vi "ex10.vi"() -> ()   [LabVIEW 2025]
panel:
  out "impairs":i32[](array[numeric])
  out "pair":i32[](array[numeric])
  in  "input":i32[][](array[numeric])
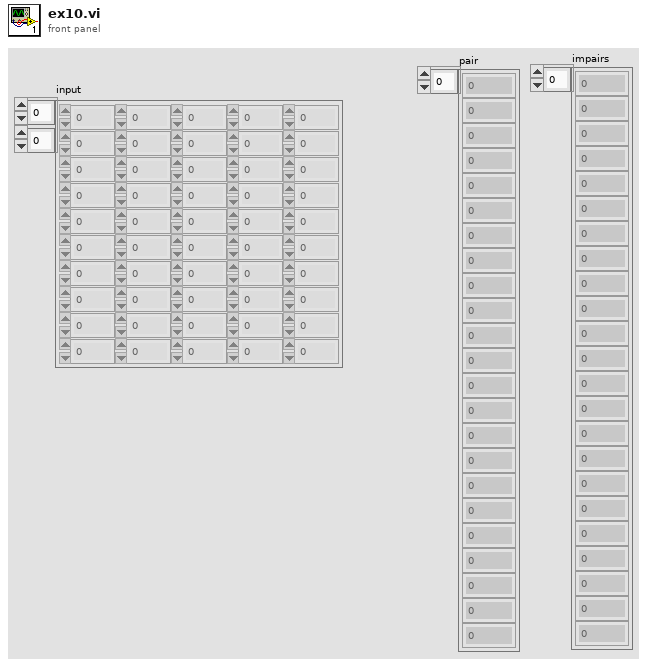
[diagram p1: front panel]
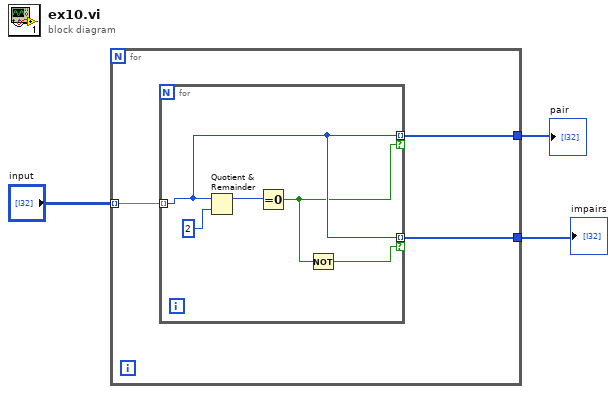
[diagram p0: block diagram]
diagram:
  n1 = for {
    tunnel: "input" -> [w6] mode=indexing
    tunnel: [w5] -> w2
    tunnel: [w4] -> w1
    n2 = for {
      tunnel: w6 -> [w9] mode=indexing
      tunnel: [w9] -> w5 mode=indexing if=w7
      tunnel: [w9] -> w4 mode=indexing if=w8
      n3 = Quotient & Remainder(x=w9, y=2) -> (x-y*floor(x/y)=w10:i32)  [unwired: 1 out]
      n4 = Equal To 0?(x=w10) -> (x = 0?=w7:bool)
      n5 = Not(x=w7) -> (.not. x?=w8:bool)
    }
  }
  "pair" <- w2
  "impairs" <- w1
